vi "Update AppInst Ring.vi"(9 "Old Value":u16, 10 "AppInst in":refnum<vi>, 11 "Ring in":refnum<vi>) -> (1 "Selection Changed?":bool, 2 "AppInst out":refnum<vi>)   [LabVIEW 2009]
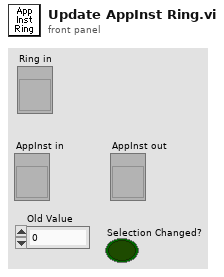
[diagram p1: front panel]
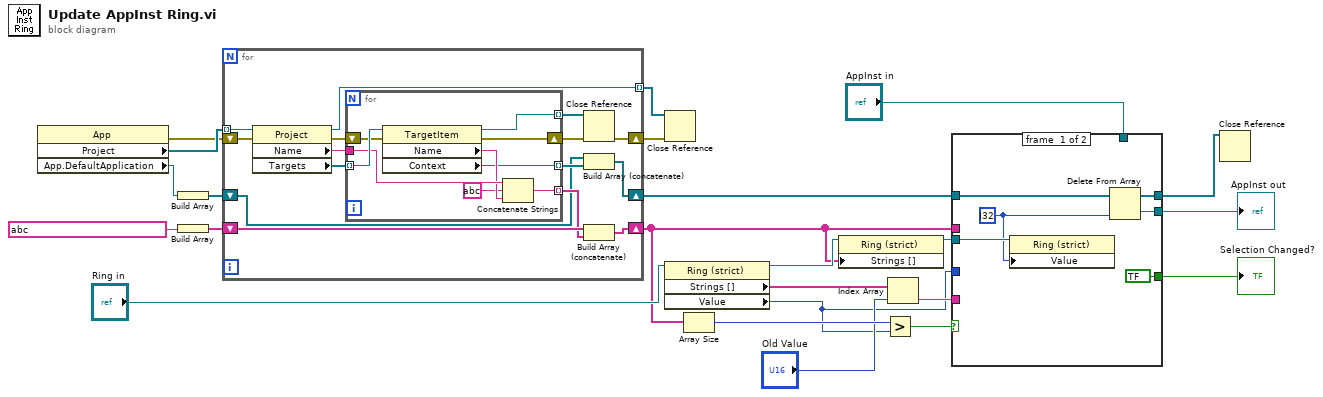
[diagram p0: block diagram]
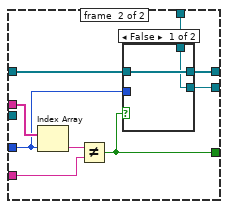
[diagram p2: hidden frame]
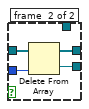
[diagram p3: hidden frame]
diagram:
  n1 = property class="App"() -> (error out=w22:errorcluster, "Project"=w23:refnum<vi>[], "App.DefaultApplication"=w4:refnum<vi>)  [unwired: 2 in, 1 out]
  n2 = Build Array(w4) -> (w20:refnum<vi>[])
  n3 = Build Array(string ?) -> (w21:string[])
  n4 = for {
    tunnel: w23 -> [w28] mode=indexing
    shift-right: [w34] -> w14
    shift-left: w21 -> [w36]
    shift-right: [w26] -> w8
    shift-left: w22 -> [w32]
    shift-right: [w30] -> w15
    shift-left: w20 -> [w29]
    tunnel: [w24] -> w7 mode=indexing
    n5 = property class="Project"(reference=w28, error in=w32) -> (reference out=w24:refnum<vi>, error out=w33:errorcluster, "Name"=w37:string, "Targets"=w38:refnum<vi>[])
    n6 = for {
      tunnel: w38 -> [w47] mode=indexing
      tunnel: w37 -> [w46]
      tunnel: [w43] -> w35 mode=indexing
      shift-right: [w40] -> w27
      shift-left: w33 -> [w42]
      tunnel: [w41] -> w31 mode=indexing
      tunnel: [w39] -> w25 mode=indexing
      n7 = property class="TargetItem"(reference=w47, error in=w42) -> (reference out=w39:refnum<vi>, error out=w40:errorcluster, "Name"=w45:string, "Context"=w41:refnum<vi>)
      n8 = Concatenate Strings(w46, string ? ("string"), w45) -> (w43:string)
    }
    n9 = Close Reference(reference=w25, error in (no error)=w27) -> (error out=w26:errorcluster)
    n10 = Build Array (concatenate)(w29, w31) -> (w30:refnum<vi>[])
    n11 = Build Array (concatenate)(w36, w35) -> (w34:string[])
  }
  n12 = Close Reference(reference=w7, error in (no error)=w8) -> ()  [unwired: 1 out]
  n13 = property class="Ring (strict)"(reference="Ring in") -> (reference out=w17:refnum<vi>, "Strings []"=w18:string[], "Value"=w1:u16)  [unwired: 1 in, 1 out]
  n14 = Array Size(array=w14) -> (size(s)=w13:i32)
  n15 = property class="Ring (strict)"(reference=w17, "Strings []"=w14) -> (reference out=w11:refnum<vi>)  [unwired: 1 in, 1 out]
  n16 = Greater?(x=w13, y=w1) -> (0:w12:bool)
  n17 = Index Array(array=w18, index="Old Value") -> (element=w5:string)
  n18 = case shown="True" w12 {
    tunnel: w14 -> [_ w62]
    tunnel: [bool ? w56] -> w16
    tunnel: w15 -> [w52 w60]
    tunnel: w1 -> [_ w59]
    tunnel: [w50 w58] -> w10
    tunnel: [w51 w57] -> w9
    tunnel: w11 -> [w49 _]
    tunnel: "AppInst in" -> [_ w55]
    tunnel: w5 -> [_ w54]
    frame #0 {
      w48 = i32 ? ("index")
      n19 = property class="Ring (strict)"(reference=w49, "Value"=w48) -> ()  [unwired: 1 in, 2 out]
      n20 = Delete From Array(array=w52, index=w48) -> (deleted portion=w50:refnum<vi>, array with subset deleted=w51:refnum<vi>[])  [unwired: 1 in]
    }
    frame #1 {
      n21 = Index Array(array=w62, index=w59) -> (element=w61:string)
      n22 = Not Equal?(x=w61, y=w54) -> (x != y?=w56:bool)
      n23 = case shown="False" w56 {
        tunnel: w60 -> [w64 w68]
        tunnel: w59 -> [_ w67]
        tunnel: [w63 w66] -> w58
        tunnel: [w64 w65] -> w57
        tunnel: w55 -> [w63 _]
        frame #0 {
        }
        frame #1 {
          n24 = Delete From Array(array=w68, index=w67) -> (deleted portion=w66:refnum<vi>, array with subset deleted=w65:refnum<vi>[])  [unwired: 1 in]
        }
      }
    }
  }
  "AppInst out" <- w10
  "Selection Changed?" <- w16
  n25 = Close Reference(reference=w9) -> ()  [unwired: 1 in, 1 out]
